vi "Compare Model dlls.vi"(8 "Error (in)":errorcluster, 10 "Model Filepath B":path, 11 "Model Filepath A":path) -> (0 "Error (out)":errorcluster)   [LabVIEW 2016]
panel:
  out "MD5 Match?":bool
  out "MD5 File B":string
  out "MD5 File A":string
  out "Model Items Added":string[](array[string])
  out "Model Items Removed":string[](array[string])
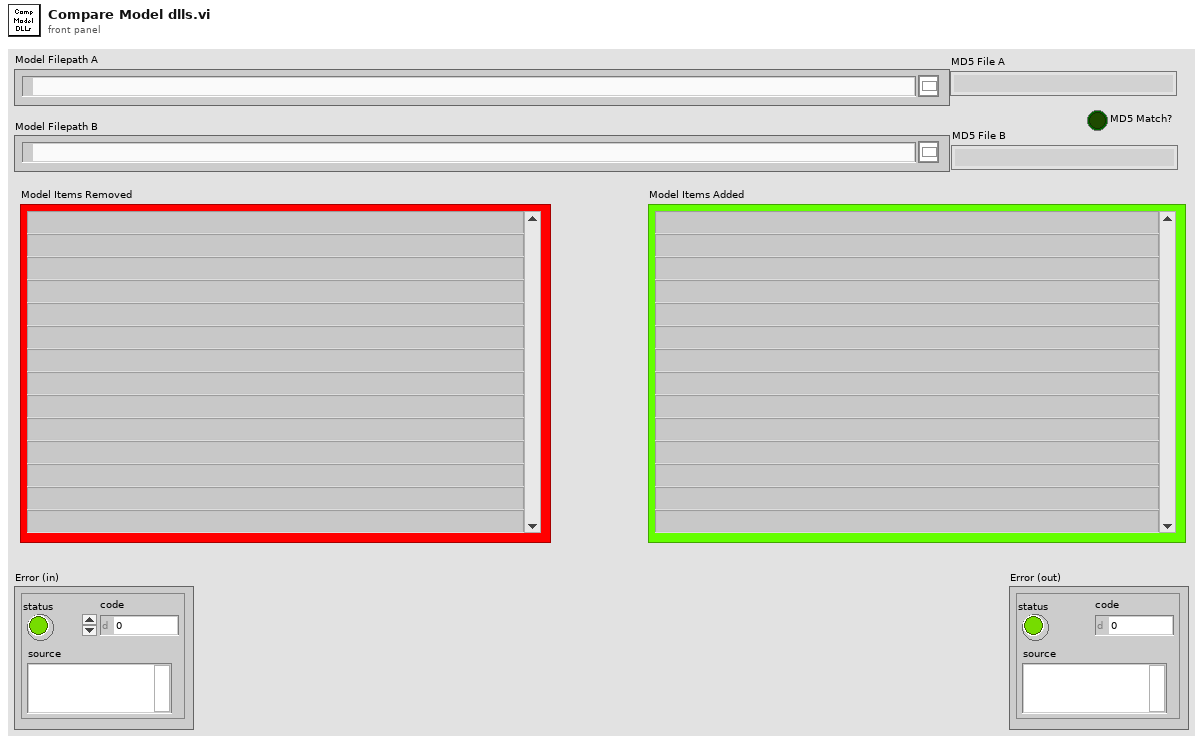
[diagram p1: front panel]
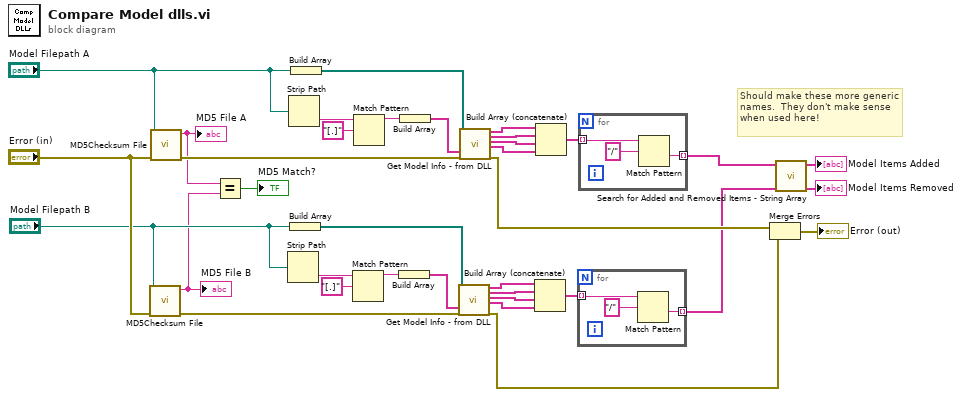
[diagram p0: block diagram]
diagram:
  # "Should make these more generic names.  They don't make sense when used here!"
  n1 = call <vilib>:"MD5Checksum File.vi"("error in (no error)"="Error (in)", "Path"="Model Filepath B") -> ("error out"=w10:errorcluster, "MD5 message-digest"=w3:string)  [unwired: 8 in]
  "MD5 File B" <- w3
  n2 = call <vilib>:"MD5Checksum File.vi"("error in (no error)"="Error (in)", "Path"="Model Filepath A") -> ("error out"=w22:errorcluster, "MD5 message-digest"=w4:string)  [unwired: 8 in]
  "MD5 File A" <- w4
  n3 = Equal?(x=w4, y=w3) -> (x = y?=→"MD5 Match?":bool)
  n4 = Strip Path(path="Model Filepath B") -> (name=w19:string)  [unwired: 1 out]
  n5 = Strip Path(path="Model Filepath A") -> (name=w34:string)  [unwired: 1 out]
  n6 = Build Array("Model Filepath B") -> (w20:path[])
  n7 = Build Array("Model Filepath A") -> (w35:path[])
  n8 = Match Pattern(string=w19, regular expression="[.]") -> (before substring=w16:string)  [unwired: 1 in, 3 out]
  n9 = Match Pattern(string=w34, regular expression="[.]") -> (before substring=w31:string)  [unwired: 1 in, 3 out]
  n10 = Build Array(w16) -> (w17:string[])
  n11 = Build Array(w31) -> (w32:string[])
  n12 = call "Get Model Info - from DLL.vi"("Model Filepaths"=w20, "Models"=w17, "Error (in)"=w10) -> ("DLL Inports"=w15:string[], "DLL Outports"=w14:string[], "DLL Parameters"=w13:string[], "DLL Signals"=w12:string[], "Error (out)"=w6:errorcluster)  [unwired: 12 in]
  n13 = call "Get Model Info - from DLL.vi"("Model Filepaths"=w35, "Models"=w32, "Error (in)"=w22) -> ("DLL Inports"=w30:string[], "DLL Outports"=w29:string[], "DLL Parameters"=w28:string[], "DLL Signals"=w27:string[], "Error (out)"=w7:errorcluster)  [unwired: 12 in]
  n14 = Build Array (concatenate)(w15, w14, w13, w12) -> (w11:string[])
  n15 = Build Array (concatenate)(w30, w29, w28, w27) -> (w23:string[])
  n16 = for {
    tunnel: w11 -> [w38] mode=indexing
    tunnel: [w36] -> w1 mode=indexing
    n17 = Match Pattern(string=w38, regular expression="/") -> (after substring=w36:string)  [unwired: 1 in, 3 out]
  }
  n18 = for {
    tunnel: w23 -> [w41] mode=indexing
    tunnel: [w39] -> w2 mode=indexing
    n19 = Match Pattern(string=w41, regular expression="/") -> (after substring=w39:string)  [unwired: 1 in, 3 out]
  }
  n20 = Merge Errors(w7, w6) -> (→"Error (out)":errorcluster)
  n21 = call "Search for Added and Removed Items - String Array.vi"("Model"=w1, "SysDef"=w2) -> ("Model Items Removed"=→"Model Items Removed":string[], "Model Items Added"=→"Model Items Added":string[])  [unwired: 8 in]
